vi "Raise Status Bar Text Changed Event.vi"(4 "user event":refnum<user-event>, 5 "Event Data":cluster{"sender":refnum<k24>, "e":refnum<k24>}, 6 "Control Ref":refnum<k24>, 7 "Event Common Data":T1) -> ()   [LabVIEW 2024, in "WebView.lvclass"]
uses:
  WebView.lvclass
  <vilib>/sklein/WebView2/Libs/Microsoft.Web.WebView2.Core.dll
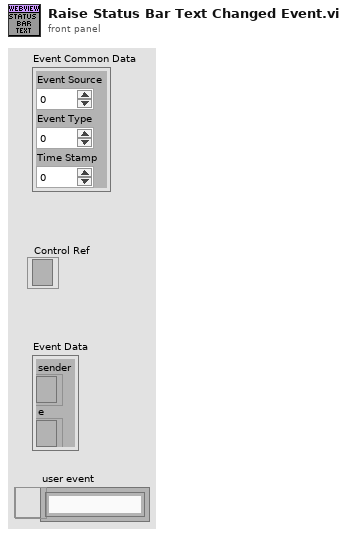
[diagram p1: front panel]
types:
  T1 = cluster{"Event Source":i32, "Event Type":u32, "Time Stamp":u32}
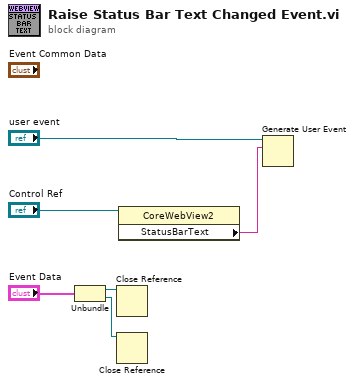
[diagram p0: block diagram]
diagram:
  n1 = Unbundle("Event Data") -> ("sender"=w3:refnum<k24>, "e"=w2:refnum<k24>)
  n2 = Close Reference(reference=w3) -> ()  [unwired: 1 in, 1 out]
  n3 = Close Reference(reference=w2) -> ()  [unwired: 1 in, 1 out]
  n4 = property class="CoreWebView2"(reference="Control Ref") -> ("StatusBarText"=w5:string)  [unwired: 1 in, 2 out]
  n5 = Generate User Event(user event="user event", event data cluster=w5) -> ()  [unwired: 2 in, 2 out]
